vi "SetTxLabelDecimation.vi"(6 "SectionBaseRate":i32, 7 "ScheduledSDI":bool, 8 "error in (no error)":errorcluster, 11 "Labels Settings In":T1[](array[typedef]) {"Words"."Param Setting"."Num Bits" min=1 max=32; "Words"."Param Setting"."Start Bit" min=8 max=31; "Words"."Block Data Refs"."Data Reference" format="%.0x"; "Label" format="%.0o"}) -> (0 "error out":errorcluster, 3 "Label Settings Out":T1[](array[typedef]) {"Words"."Param Setting"."Num Bits" min=1 max=32; "Words"."Param Setting"."Start Bit" min=8 max=31; "Words"."Block Data Refs"."Data Reference" format="%.0x"; "Label" format="%.0o"})   [LabVIEW 2017]
uses:
  Shared/Controls and Global/Label.ctl
  Shared/Ballard Arinc-429 Shared.lvlib
  Shared/Controls and Global/transferPeriod.ctl
  <vilib>/NI Veristand/Custom Device API/Data Reference.ctl
  <vilib>/NI Veristand/Custom Device API/Custom Device API.lvlib
  <vilib>/NI Veristand/Custom Device API/Block Data Reference.ctl
  Shared/Controls and Global/Start Bit.ctl
  Shared/Controls and Global/Number of Bits.ctl
  RT Controls/Driver Data.ctl
  RT Controls/RT Label Settings.ctl
  Ballard Arinc-429 Engine.lvlib
  RT Controls/RT Param Setting.ctl
  RT Controls/RT Word Settings.ctl
  Shared/Controls and Global/TransferType.ctl
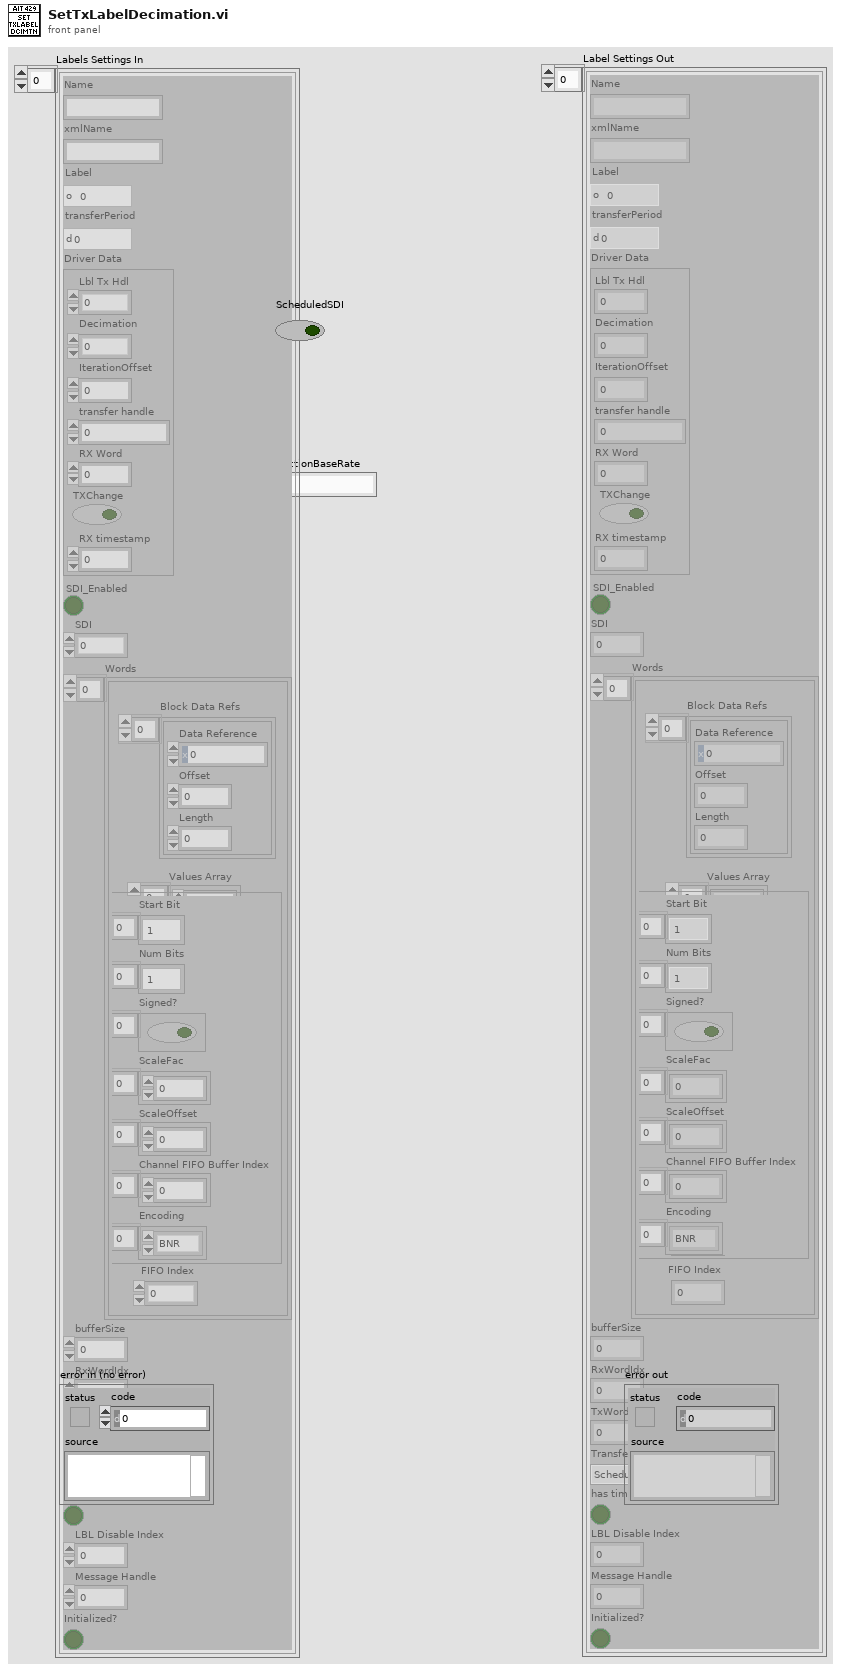
[diagram p1: front panel]
types:
  T1 = typedef "Ballard Arinc-429 Engine.lvlib/RT Label Settings.ctl" = cluster{"Name":string, "xmlName":string, "Label":T2, "transferPeriod":T3, "Driver Data":T4, "SDI_Enabled":bool, "SDI":u8, "Words":T5[], "bufferSize":u32, "RxWordIdx":i32, "TxWordIdx":i32, "TransferType":T11, "has timestamp?":bool, "LBL Disable Index":i32, "Message Handle":u64, "Initialized?":bool}
  T2 = typedef "Ballard Arinc-429 Shared.lvlib/Label.ctl" = u8
  T3 = typedef "Ballard Arinc-429 Shared.lvlib/transferPeriod.ctl" = u32
  T4 = typedef "Driver Data.ctl" = cluster{"Lbl Tx Hdl":u32, "Decimation":i32, "IterationOffset":i32, "transfer handle":u32, "RX Word":u32, "TXChange":bool, "RX timestamp":dbl}
  T5 = typedef "Ballard Arinc-429 Engine.lvlib/RT Word Settings.ctl" = cluster{"Block Data Refs":T6[], "Values Array":dbl[], "Length":i32, "FIFO Index":i32, "Param Setting":T8}
  T6 = typedef "Custom Device API.lvlib/Block Data Reference.ctl" = cluster{"Data Reference":T7, "Offset":u64, "Length":u64}
  T7 = typedef "Custom Device API.lvlib/Data Reference.ctl" = i32
  T8 = typedef "Ballard Arinc-429 Engine.lvlib/RT Param Setting.ctl" = cluster{"Start Bit":T9[], "Num Bits":T10[], "Signed?":bool[], "ScaleFac":dbl[], "ScaleOffset":dbl[], "Channel FIFO Buffer Index":i32[], "Encoding":enum16{"BNR", "BCD", "Discrete"}[]}
  T9 = typedef "Ballard Arinc-429 Shared.lvlib/Start Bit.ctl" = i32
  T10 = typedef "Ballard Arinc-429 Shared.lvlib/Number of Bits.ctl" = i32
  T11 = typedef "Ballard Arinc-429 Shared.lvlib/TransferType.ctl" = enum16{"ScheduledLabel", "Acyclic", "Block", "Strobe"}
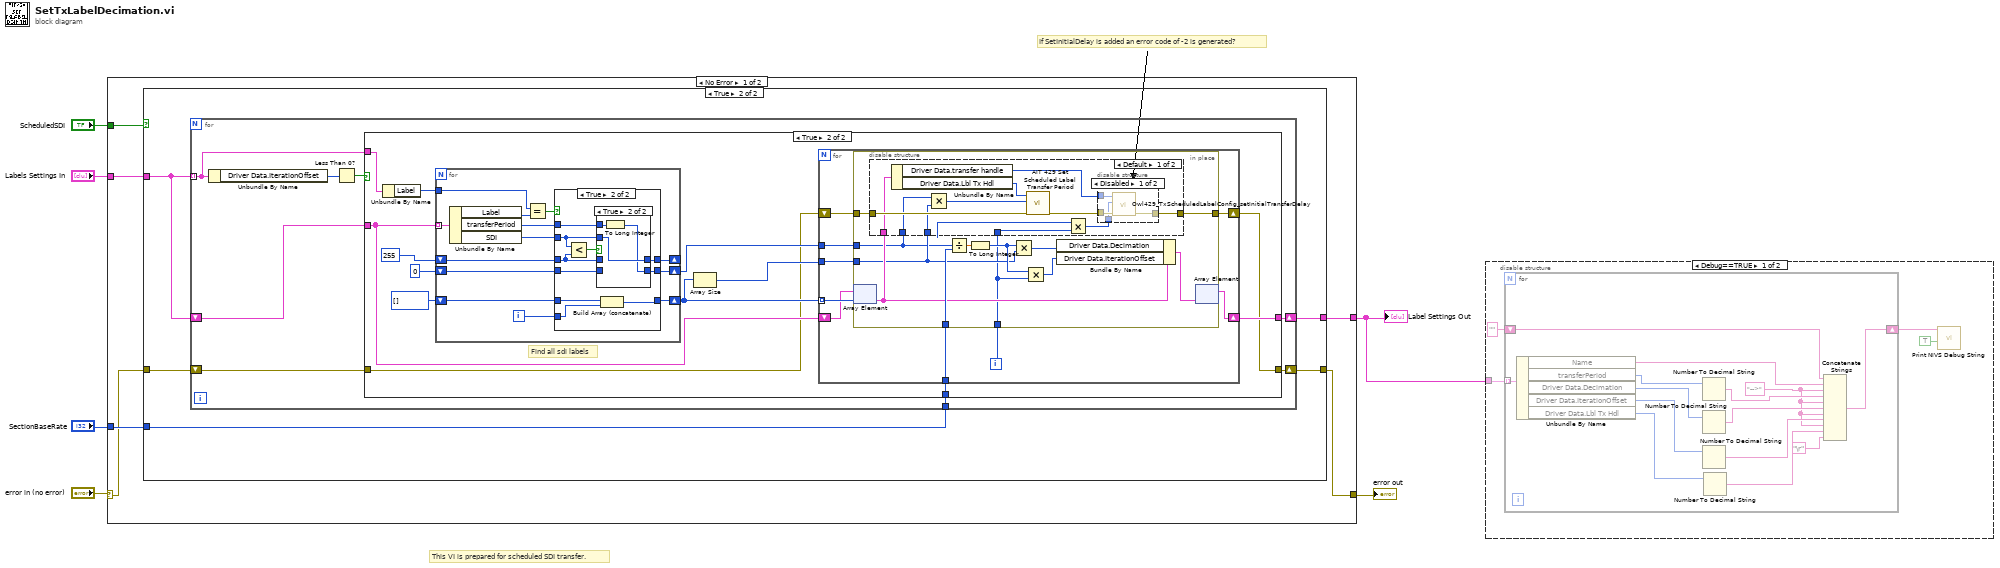
[diagram p0: block diagram]
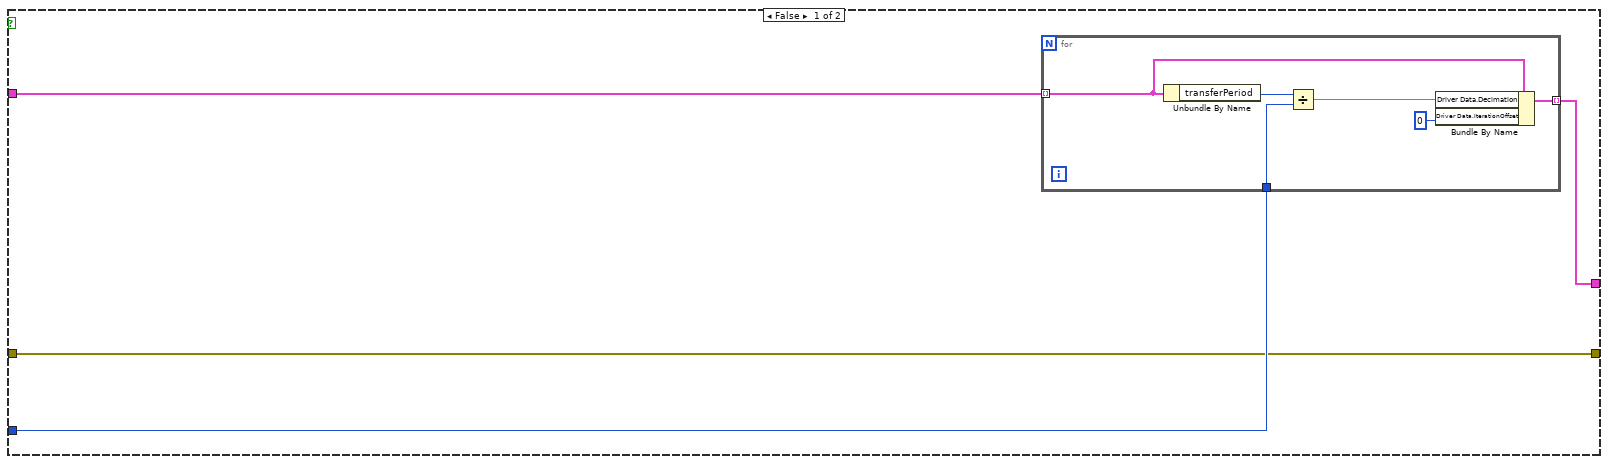
[diagram p3: hidden frame]
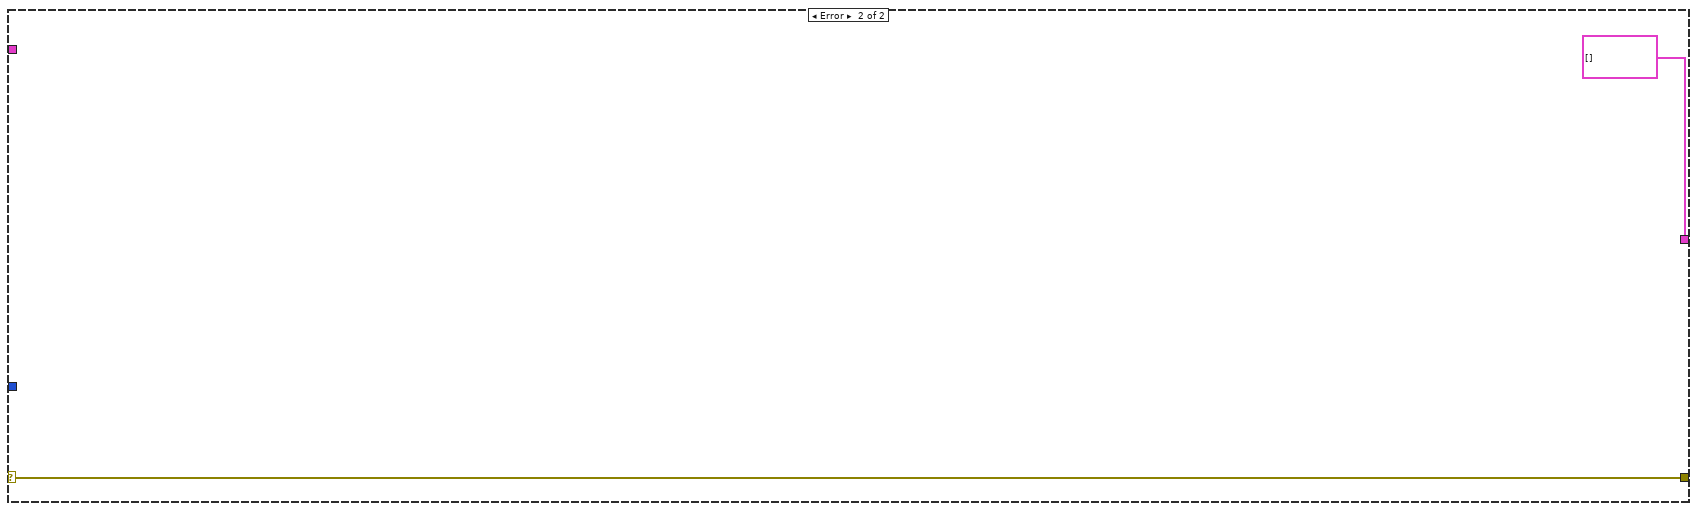
[diagram p9: hidden frame]
diagram:
  # "If SetInitialDelay is added an error code of -2 is generated?"
  # "This VI is prepared for scheduled SDI transfer."
  n1 = case shown="No Error" "error in (no error)" {
    selector: "error in (no error)" -> [w7 w120]
    tunnel: [w12 T1[] []] -> w1
    tunnel: "SectionBaseRate" -> [w11 _]
    tunnel: [w8 w120] -> w4
    tunnel: "Labels Settings In" -> [w10 _]
    tunnel: "ScheduledSDI" -> [w9 _]
    frame No Error {
      n2 = case shown="True" w9 {
        tunnel: [w16 w26] -> w12
        tunnel: w11 -> [w14 w23]
        tunnel: w10 -> [w15 w27]
        tunnel: [w13 w25] -> w8
        tunnel: w7 -> [w13 w24]
        frame False {
          n3 = for {
            tunnel: w15 -> [w20] mode=indexing
            tunnel: w14 -> [w21]
            tunnel: [w18] -> w16 mode=indexing
            n4 = Unbundle By Name(w20) -> ("transferPeriod"=w22:T3)
            n5 = Divide(x=w22, y=w21) -> (x/y=w19:dbl)
            n6 = Bundle By Name(cluster=w20, "Driver Data.Decimation"=w19, "Driver Data.IterationOffset"=0) -> (w18:T1)
          }
        }
        frame True {
          n7 = for {
            tunnel: w27 -> [w33] mode=indexing
            tunnel: w23 -> [w35]
            shift-right: [w30] -> w26
            shift-left: w27 -> [w34]
            shift-right: [w28] -> w25
            shift-left: w24 -> [w29]
            n8 = Unbundle By Name(w33) -> ("Driver Data.IterationOffset"=w32:i32)
            n9 = Less Than 0?(x=w32) -> (x < 0?=w31:bool)
            n10 = case shown="True" w31 {
              tunnel: w35 -> [_ w42]
              tunnel: w34 -> [w37 w44]
              tunnel: w33 -> [_ w50]
              tunnel: [w37 w41] -> w30
              tunnel: w29 -> [w36 w39]
              tunnel: [w36 w38] -> w28
              frame False {
              }
              frame True {
                # "Find all sdi labels"
                n11 = Unbundle By Name(w50) -> ("Label"=w49:T2)
                n12 = for {
                  shift-right: [w96] -> w45
                  shift-left: i32[] [] -> [w97]
                  tunnel: w44 -> [w101] mode=indexing
                  tunnel: w49 -> [w100]
                  shift-right: [w90] -> w43
                  shift-left: 0 -> [w92]
                  shift-right: [w89] -> _
                  shift-left: u8 255 -> [w91]
                  i -> [w95]
                  n13 = Unbundle By Name(w101) -> ("Label"=w99:T2, "transferPeriod"=w94:T3, "SDI"=w93:u8)
                  n14 = Equal?(x=w100, y=w99) -> (x = y?=w98:bool)
                  n15 = case shown="True" w98 {
                    tunnel: w97 -> [w104 w114]
                    tunnel: [w104 w112] -> w96
                    tunnel: w95 -> [_ w113]
                    tunnel: w94 -> [_ w109]
                    tunnel: w93 -> [_ w106]
                    tunnel: w92 -> [w102 w110]
                    tunnel: w91 -> [w103 w107]
                    tunnel: [w102 w108] -> w90
                    tunnel: [w103 w105] -> w89
                    frame False {
                    }
                    frame True {
                      n16 = Less?(x=w106, y=w107) -> (x < y?=w111:bool)
                      n17 = case shown="True" w111 {
                        tunnel: w110 -> [w115 _]
                        tunnel: w109 -> [_ w119]
                        tunnel: [w115 w117] -> w108
                        tunnel: w107 -> [w116 _]
                        tunnel: w106 -> [_ w118]
                        tunnel: [w116 w118] -> w105
                        frame False {
                        }
                        frame True {
                          n18 = To Long Integer(number=w119) -> (32bit integer=w117:i32)
                        }
                      }
                      n19 = Build Array (concatenate)(w114, w113) -> (w112:i32[])
                    }
                  }
                }
                n20 = Array Size(array=w45) -> (size(s)=w40:i32)
                n21 = for {
                  tunnel: w45 -> [w59] mode=indexing
                  tunnel: w40 -> [w53]
                  tunnel: w43 -> [w56]
                  tunnel: w42 -> [w55]
                  shift-right: [w57] -> w41
                  shift-left: w44 -> [w58]
                  shift-right: [w51] -> w38
                  shift-left: w39 -> [w52]
                  i -> [w54]
                  n22 = in-place {
                    in-place-border: w56 -> [w61]
                    in-place-border: w55 -> [w70]
                    in-place-border: w54 -> [w60]
                    in-place-border: w53 -> [w62]
                    in-place-border: w52 -> [w65]
                    in-place-border: [w64] -> w51
                    n23 = in-place-array #1(w58, w59) -> (w63:T1)
                    n24 = disable-structure shown="Default" {
                      disable-tunnel: w65 -> [w82 w88]
                      disable-tunnel: [w80 w88] -> w64
                      disable-tunnel: w63 -> [w79 _]
                      disable-tunnel: w62 -> [w78 _]
                      disable-tunnel: w61 -> [w76 _]
                      disable-tunnel: w60 -> [w74 _]
                      frame condition #0 (active) {
                        n25 = Unbundle By Name(w79) -> ("Driver Data.transfer handle"=w72:u32, "Driver Data.Lbl Tx Hdl"=w73:u32)
                        n26 = Multiply(x=w76, y=w78) -> (x*y=w77:i32)
                        n27 = call <instrlib>:"AIT 429 Set Scheduled Label Transfer Period.vi"("error in (no error)"=w82, "transfer period"=w77, "scheduled label handle"=w73) -> ("error out"=w81:errorcluster)  [unwired: 7 in, 1 out]
                        n28 = Multiply(x=w76, y=w74) -> (x*y=w75:i32)
                        n29 = disable-structure shown="Disabled" {
                          disable-tunnel: w81 -> [w86 w87]
                          disable-tunnel: [w85 w87] -> w80
                          disable-tunnel: w75 -> [w84 _]
                          disable-tunnel: w72 -> [w83 _]
                          frame Disabled {
                            n30 = call <userlib>:"Owl429_TxScheduledLabelConfig_setInitialTransferDelay.vi"("error in (no error)"=w86, "delay"=w84, "label config handle"=w83) -> ("error out"=w85:errorcluster)  [unwired: 7 in, 1 out]
                          }
                          frame Enabled {
                          }
                        }
                      }
                      frame condition #1 {
                      }
                    }
                    n31 = Divide(x=w61, y=w70) -> (x/y=w67:dbl)
                    n32 = To Long Integer(number=w67) -> (32bit integer=w66:i32)
                    n33 = Multiply(x=w66, y=w62) -> (x*y=w68:i32)
                    n34 = Multiply(x=w66, y=w60) -> (x*y=w69:i32)
                    n35 = Bundle By Name(cluster=w63, "Driver Data.Decimation"=w68, "Driver Data.IterationOffset"=w69) -> (w71:T1)
                    n36 = in-place-array #1(w71) -> (w57:T1[])  [unwired: 1 out]
                  }
                }
              }
            }
          }
        }
      }
    }
    frame Error {
    }
  }
  "Label Settings Out" <- w1
  "error out" <- w4
  n37 = disable-structure shown="Debug==TRUE" {
    disable-tunnel: w1 -> [w125 _]
    frame condition #0 {
      n38 = for {
        tunnel: w125 -> [w139] mode=indexing
        shift-right: [w131] -> w123
        shift-left: "" -> [w130]
        w127 = "-->" ("string")
        n39 = Unbundle By Name(w139) -> ("Name"=w135:string, "transferPeriod"=w138:T3, "Driver Data.Decimation"=w137:i32, "Driver Data.IterationOffset"=w136:i32, "Driver Data.Lbl Tx Hdl"=w129:u32)
        n40 = Number To Decimal String(number=w138) -> (decimal integer string=w134:string)  [unwired: 1 in]
        n41 = Number To Decimal String(number=w137) -> (decimal integer string=w133:string)  [unwired: 1 in]
        n42 = Number To Decimal String(number=w136) -> (decimal integer string=w132:string)  [unwired: 1 in]
        n43 = Number To Decimal String(number=w129) -> (decimal integer string=w126:string)  [unwired: 1 in]
        n44 = Concatenate Strings(w130, w135, w127, w134, w127, w133, w127, w132, w127, w126, "\r") -> (w131:string)
      }
      n45 = call "Print NIVS Debug String.vi"("Add to NIVS Log FIle? (T)"=TRUE, "Debug String"=w123) -> ()  [unwired: 8 in, 1 out]
    }
    frame condition #1 (active) {
    }
  }
